vi "Command - extract tokens.vi"(5 "Cmd string":string="power -10 0") -> (0 "N arg":u8=2, 1 "Arguments":string[](array[string])=["0", "10"], 2 "Command":string="power")   [LabVIEW 2019]
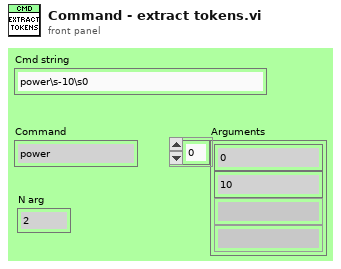
[diagram p1: front panel]
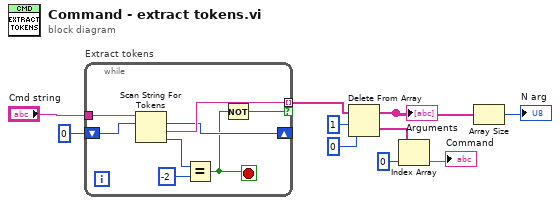
[diagram p0: block diagram]
diagram:
  n1 = while "Extract tokens" {
    tunnel: "Cmd string" -> [w18]
    shift-right: [w13] -> _
    shift-left: 0 -> [w17]
    tunnel: [w14] -> w6 mode=indexing if=w12
    stop <- w11 stop-if-true
    n2 = Scan String For Tokens(8:w17, 9:w18) -> (0:w15:i32, 1:w14:string, 2:w13:i32)  [unwired: 4 in, 1 out]
    n3 = Equal?(x=w15, y=-2) -> (x = y?=w11:bool)
    n4 = Not(x=w11) -> (.not. x?=w12:bool)
  }
  n5 = Delete From Array(array=w6, length=1, index=0) -> (deleted portion=w5:string[], array with subset deleted=w2:string[])
  "Arguments" <- w2
  n6 = Index Array(array=w5, index=0) -> (element=→"Command":string)
  n7 = Array Size(array=w2) -> (size(s)=→"N arg":i32)
